vi "BIO_read_low_level.vi"(8 "error in (no error)":errorcluster, 10 "bytes to read":i32=1024, 11 "BIO in":refnum<class "BIO.lvclass">) -> (0 "error out":errorcluster, 1 "buf":string, 2 "return type":i32, 3 "BIO out":refnum<class "BIO.lvclass">)   [LabVIEW 2013, in "SSL_Lib.lvlib" / "BIO.lvclass"]
uses:
  BIO.lvclass
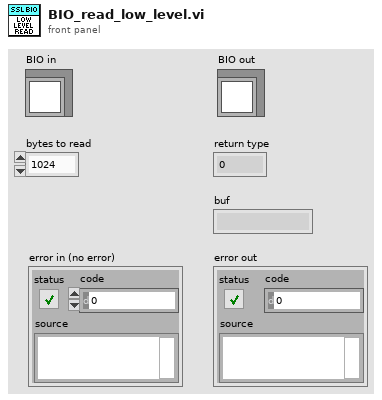
[diagram p1: front panel]
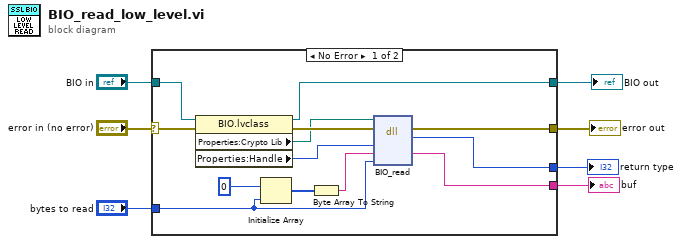
[diagram p0: block diagram]
diagram:
  n1 = case shown="No Error" "error in (no error)" {
    selector: "error in (no error)" -> [w17 w21]
    tunnel: [w20 w21] -> w7
    tunnel: [w19 _] -> w6
    tunnel: "bytes to read" -> [w10 _]
    tunnel: [w18 _] -> w4
    tunnel: "BIO in" -> [w15 w22]
    tunnel: [w13 w22] -> w1
    frame No Error {
      n2 = property class="BIO.lvclass"(reference=w15, error in=w17) -> (reference out=w13:refnum<class "BIO.lvclass">, error out=w16:errorcluster, "Properties:Crypto Lib"=w12:path, "Properties:Handle"=w14:u64)
      n3 = Initialize Array(u8 0, w10) -> (w9:u8[])
      n4 = Byte Array To String(unsigned byte array=w9) -> (string=w8:string)
      n5 = dll-call lib="C:/Program Files (x86)/National Instruments/Shared/nissl/NIlibeay32.dll" fn="BIO_read"(path in=w12, error in=w16, "BIO"=w14, "buf"=w8, "len"=w10) -> (error out=w20:errorcluster, "return type"=w19:i32, "buf"=w18:string)  [unwired: 3 in, 1 out]
    }
    frame Error {
    }
  }
  "error out" <- w7
  "return type" <- w6
  "buf" <- w4
  "BIO out" <- w1
